vi "PI_controller_dt.vi"(4 "dv in":bool, 6 "xy_diff_in":fxp<+/-,16,8>, 8 "scan_int":fxp<+,16,2>=0.00201416015625, 9 "write_first_centroid":bool, 10 "proportional":fxp<+,16,2>, 11 "Intmult":fxp<+/-,16,12>) -> (2 "xydiffvalid":bool, 3 "xydiff_out":fxp<+/-,16,8>)   [LabVIEW 2020]
uses:
  <vilib>/rvi/FXPMathLib/FxpMul/XNode/nifxpmath_Multiplier.xnode
  <vilib>/rvi/FXPMathLib/FxpAdd/XNode/nifxpmath_Add.xnode
  <vilib>/rvi/FXPMathLib/sim/FxpSim.dll
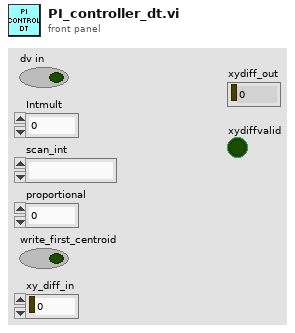
[diagram p1: front panel]
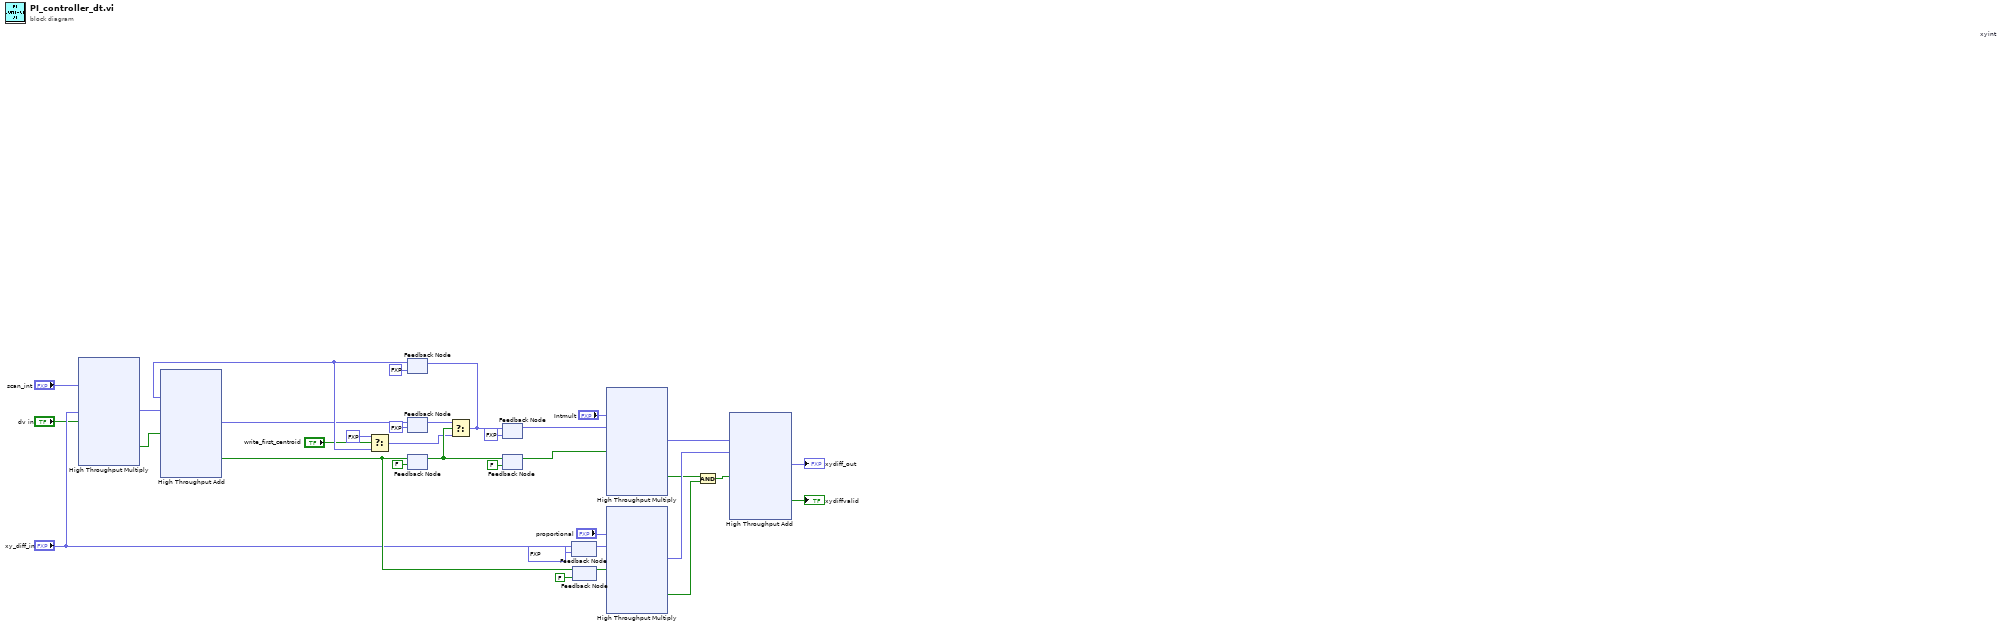
[diagram p0: block diagram]
diagram:
  n1 = xnode ("High Throughput Multiply")("x"="scan_int", "y"="xy_diff_in", "input valid"="dv in") -> ("x*y"=w11:fxp<+/-,16,2>, "output valid"=w9:bool)  [unwired: 1 in, 1 out]
  n2 = feedback #1(fxp<+/-,21,8> data[17B] ("t")) -> (w18:fxp<+/-,21,8>)
  n3 = xnode ("High Throughput Add")("x"=w18, "y"=w11, "input valid"=w9) -> ("x+y"=w15:fxp<+/-,16,3>, "output valid"=w25:bool)  [unwired: 1 in, 1 out]
  n4 = Select(t=fxp<+/-,21,8> data[17B], s="write_first_centroid", f=w18) -> (s? t:f=w14:fxp<+/-,21,8>)
  n5 = feedback #2(fxp<+/-,16,3> data[17B] ("x+y")) -> (w16:fxp<+/-,16,3>)
  n6 = feedback-in #2(w15) -> ()
  n7 = feedback #3(FALSE ("dv in")) -> (w20:bool)
  n8 = feedback-in #3(w25) -> ()
  n9 = Select(t=w16, s=w20, f=w14) -> (s? t:f=w2:fxp<+/-,21,8>)
  n10 = feedback-in #1(w2) -> ()
  n11 = feedback #4 "xyint"(fxp<+/-,21,8> data[17B] ("t")) -> (w1:fxp<+/-,21,8>)
  n12 = feedback-in #4(w2) -> ()
  n13 = feedback #5(FALSE ("dv in")) -> (w23:bool)
  n14 = feedback-in #5(w20) -> ()
  n15 = feedback #6(fxp<+/-,16,8>[] data[68B]) -> (w22:fxp<+/-,16,8>)
  n16 = feedback-in #6("xy_diff_in") -> ()
  n17 = feedback #7(FALSE ("output valid")) -> (w24:bool)
  n18 = feedback-in #7(w25) -> ()
  n19 = xnode ("High Throughput Multiply")("x"="Intmult", "y"=w1, "input valid"=w23) -> ("x*y"=w31:fxp<+/-,16,8>, "output valid"=w28:bool)  [unwired: 1 in, 1 out]
  n20 = xnode ("High Throughput Multiply")("x"="proportional", "y"=w22, "input valid"=w24) -> ("x*y"=w32:fxp<+/-,16,8>, "output valid"=w29:bool)  [unwired: 1 in, 1 out]
  n21 = And(x=w28, y=w29) -> (x .and. y?=w30:bool)
  n22 = xnode ("High Throughput Add")("x"=w31, "y"=w32, "input valid"=w30) -> ("x+y"=→"xydiff_out":fxp<+/-,16,8>, "output valid"=→"xydiffvalid":bool)  [unwired: 1 in, 1 out]
